vi "SENS_SEGM_DEL.vi"(0 "VISA IN":refnum<visa-resource-name>, 1 "Segment":i32, 5 "error in":errorcluster, 7 "Channel":i32) -> (14 "VISA Out":refnum<visa-resource-name>, 19 "error out":errorcluster)   [LabVIEW 2018, in "PNA-X.lvlib"]
doc: "SENSe<cnum>:SEGMent<snum>:DELete \n(Write-only) Deletes the specified sweep segment. When ALL segments are deleted, Sweep Mode \n(SENS:SWE:MODE) is automatically set to Linear because there are no segments to sweep. \n<cnum> Any existing channel number. If unspecified, value is set to 1 \n<snum> Number of the segment to delete. If unspecified, value is set to 1 \nExamples SENS:SEGM:DEL \nsense2:segment2:delete \nQuery Syntax Not applicable \nDefault Not Applicable \n1807"
uses:
  PNA-X.lvlib
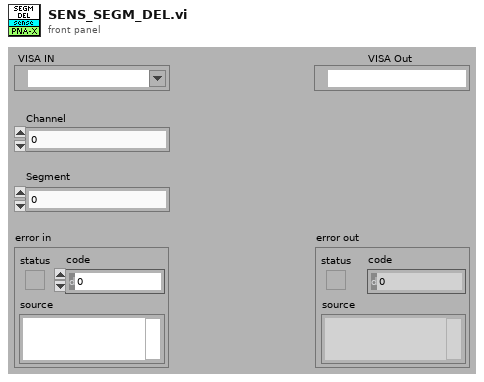
[diagram p1: front panel]
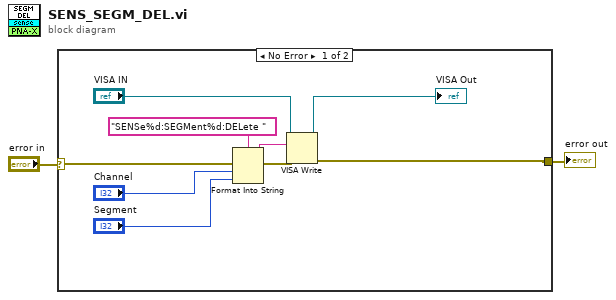
[diagram p0: block diagram]
diagram:
  n1 = case shown="No Error" "error in" {
    selector: "error in" -> [w11 w12]
    tunnel: [w6 w12] -> w1
    frame No Error {
      n2 = Format Into String(format string="SENSe%d:SEGMent%d:DELete " ("Cmdline"), error in=w11, "Channel", "Segment") -> (resulting string=w9:string, error out=w10:errorcluster)  [unwired: 1 in]
      n3 = VISA Write(VISA resource name="VISA IN", write buffer=w9, error in (no error)=w10) -> (VISA resource name out=→"VISA Out":refnum<visa-resource-name>, error out=w6:errorcluster)  [unwired: 1 out]
    }
    frame Error {
    }
  }
  "error out" <- w1
